vi "Continuous Volume Demo.vi"() -> ()   [LabVIEW 2012]
uses:
  LabVIEW/user.lib/SpectralRadar.llb/Data Analyzation Selection.ctl
  LabVIEW/user.lib/SpectralRadar.llb/Device Camera Preset Selection.ctl
  LabVIEW/user.lib/SpectralRadar.llb/Processing Flag Selection.ctl
  LabVIEW/user.lib/SpectralRadar.llb/Normal Direction Selection.ctl
  LabVIEW/user.lib/SpectralRadar.llb/set Apodized Spectrum Output.vi
  LabVIEW/user.lib/SpectralRadar.llb/set Scan Output.vi
  LabVIEW/user.lib/SpectralRadar.llb/display Data 2D.vi
  LabVIEW/user.lib/SpectralRadar.llb/OCT Device.lvclass
  LabVIEW/user.lib/SpectralRadar.llb/Probe.lvclass
  LabVIEW/user.lib/SpectralRadar.llb/Processing.lvclass
  LabVIEW/user.lib/SpectralRadar.llb/Raw Data.lvclass
  LabVIEW/user.lib/SpectralRadar.llb/Data.lvclass
  LabVIEW/user.lib/SpectralRadar.llb/Scan Pattern.lvclass
panel:
  in  "Slice vs. Process":bool
  in  "Data Analyzation Selection":T1
  out "B-Scan Data":dbl[][](graph)
  in  "Index":i32(slide) min=0 max=1023 step=1 scale=0.0..1023.0
  in  "stop":bool
  out "En-Face Data":dbl[][](graph)
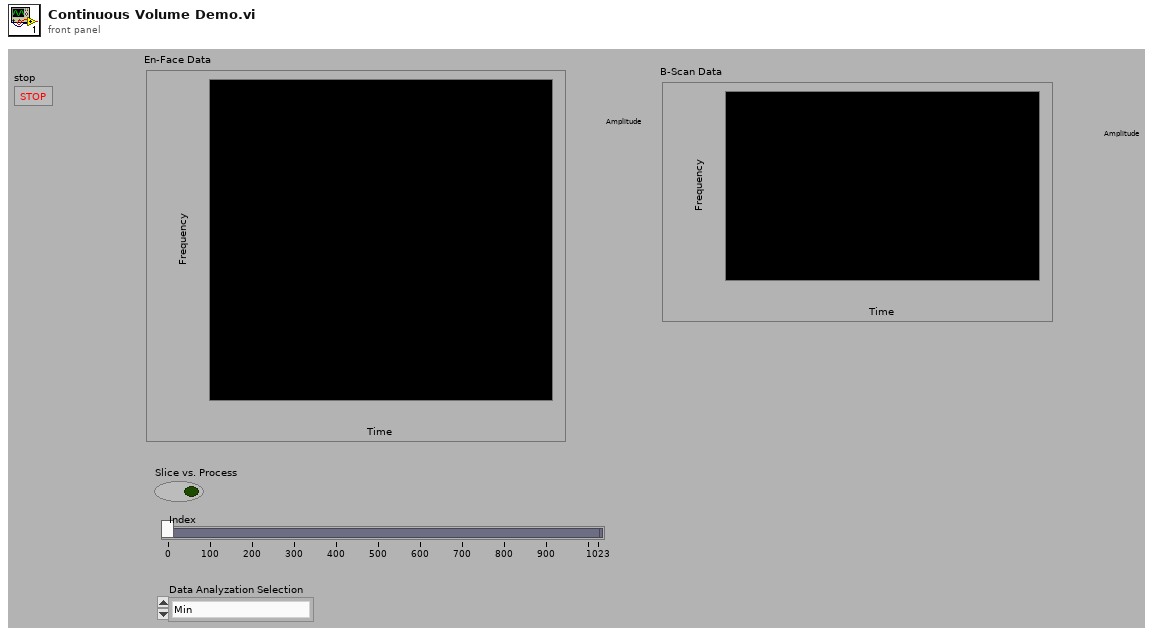
[diagram p1: front panel]
types:
  T1 = typedef "Data.lvclass/Data Analyzation Selection.ctl" = enum16{"Min", "Mean", "Max"}
  T2 = typedef "Processing.lvclass/Processing Flag Selection.ctl" = enum16{"Use Offset Errors", "Remove DC Spectrum", "Remove Advanced DC Spectrum", "Use Apodization", "Use Scan For Apodization", "Filter Undersampled Signals", "Use Dispersion Compensation", "Use Dechirp", "Use Extended Adjust", "Full Range Output", "Filter DC", "Autocorrelation Compensation", "DEFR", "Only Windowing", "Remove Fixed Pattern"}
  T3 = typedef "OCT Device.lvclass/Device Camera Preset Selection.ctl" = enum16{"Default", "Preset 1", "Preset 2", "Preset 3"}
  T4 = enum16{"Asynchronous Continuous", "Asynchronous Finite", "Synchronous"}
  T5 = typedef "Data.lvclass/Normal Direction Selection.ctl" = enum16{"Direction 1", "Direction 2", "Direction 3"}
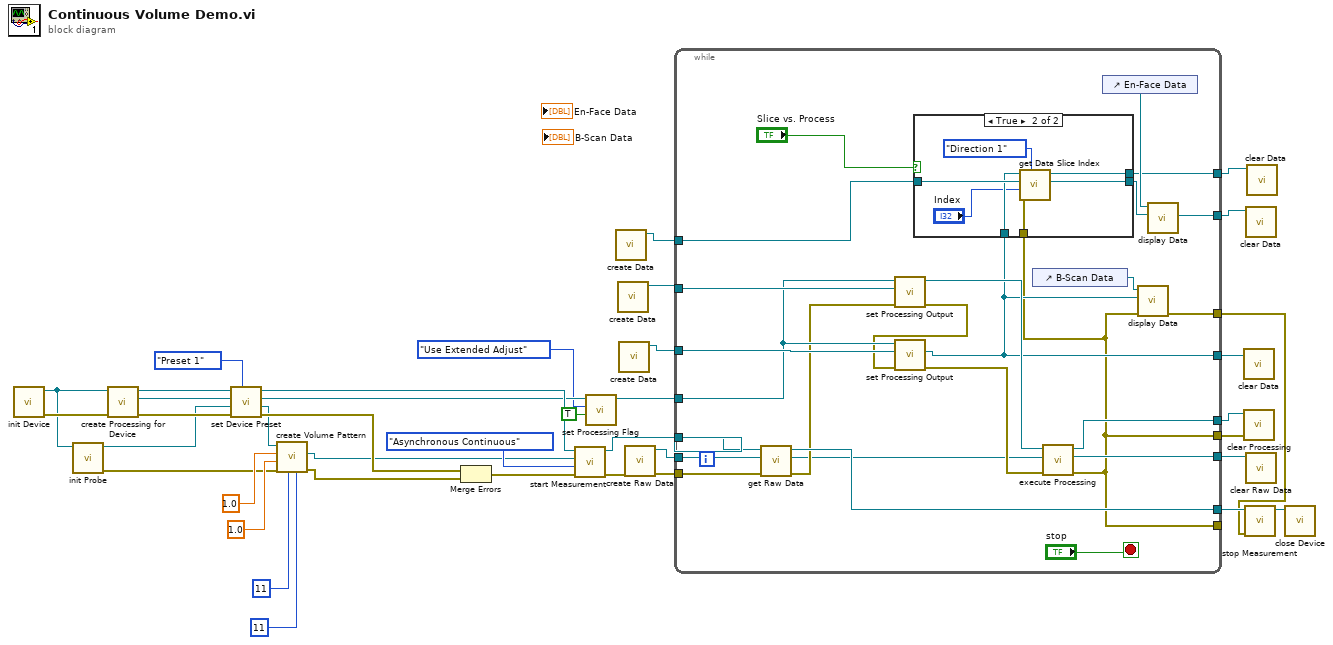
[diagram p0: block diagram]
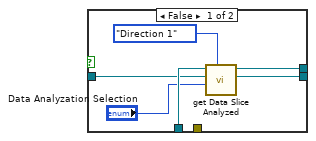
[diagram p2: hidden frame]
diagram:
  n1 = call "init Device.vi"() -> ("error out"=w38:errorcluster, "OCTDevice"=w30:refnum<class "OCT Device.lvclass">)  [unwired: 6 in]
  n2 = call "init Probe.vi"("OCT Device"=w30) -> ("error out"=w16:errorcluster, "GalvoControl"=w25:refnum<class "Probe.lvclass">)  [unwired: 5 in]
  n3 = call "create Processing for Device.vi"("error in (no error)"=w38, "OCTDevice"=w30) -> ("error out"=w35:errorcluster, "Processing"=w23:refnum<class "Processing.lvclass">, "OCTDevice"=w26:refnum<class "OCT Device.lvclass">)  [unwired: 3 in]
  n4 = call "set Device Preset.vi"("Numeric"=Device_Camera_Preset_Selection."Preset 1" ("Device Camera Preset Selection"), "Probe"=w25, "Processing"=w23, "OCTDevice"=w26) -> ("Probe 2"=w21:refnum<class "Probe.lvclass">, "Processing"=w13:refnum<class "Processing.lvclass">, "OCTDevice out"=w24:refnum<class "OCT Device.lvclass">)  [unwired: 2 in, 1 out]
  n5 = call "create Volume Pattern.vi"("Size Y"=11, "Size X"=11, "error in (no error)"=w16, "Range Y"=1.0, "Range X"=1.0, "Probe"=w21) -> ("error out"=w15:errorcluster, "Scan Pattern"=w14:refnum<class "Scan Pattern.lvclass">)  [unwired: 1 in, 1 out]
  n6 = Merge Errors(w35, w15) -> (w36:errorcluster)
  n7 = call "start Measurement.vi"("error in (no error)"=w36, "Acquisition Type"=T4."Asynchronous Continuous", "Scan Pattern"=w14, "OCTDevice"=w24) -> ("error out"=w33:errorcluster, "OCTDevice"=w27:refnum<class "OCT Device.lvclass">)  [unwired: 1 in, 1 out]
  n8 = call "set Processing Flag.vi"("Flag"=TRUE, "Processing Flag Selection"=Processing_Flag_Selection."Use Extended Adjust", "Processing"=w13) -> ("Processing"=w12:refnum<class "Processing.lvclass">)  [unwired: 3 in, 1 out]
  n9 = call "create Data.vi"() -> ("Data"=w1:refnum<class "Data.lvclass">)  [unwired: 6 in, 1 out]
  n10 = call "create Data.vi"() -> ("Data"=w2:refnum<class "Data.lvclass">)  [unwired: 6 in, 1 out]
  n11 = call "create Data.vi"() -> ("Data"=w3:refnum<class "Data.lvclass">)  [unwired: 6 in, 1 out]
  n12 = call "create Raw Data.vi"("error in (no error)"=w33) -> ("error out"=w32:errorcluster, "Raw Data"=w34:refnum<class "Raw Data.lvclass">)  [unwired: 5 in]
  n13 = while {
    tunnel: w34 -> [w62]
    tunnel: w27 -> [w63]
    tunnel: w32 -> [w61]
    tunnel: w12 -> [w58]
    tunnel: w3 -> [w60]
    tunnel: w2 -> [w59]
    tunnel: [w53] -> w31
    tunnel: [w52] -> w8
    tunnel: [w42] -> w6
    tunnel: [w51] -> w29
    tunnel: [w41] -> w7
    tunnel: [w41] -> _
    tunnel: w1 -> [w47]
    tunnel: [w46] -> w5
    tunnel: [w44] -> w4
    tunnel: [w39] -> w9
    stop <- "stop" stop-if-true
    n14 = call "get Raw Data.vi"("error in (no error)"=w61, "RawData in"=w62, "OCTDevice in"=w63) -> ("error out"=w50:errorcluster, "RawData out"=w48:refnum<class "Raw Data.lvclass">, "OCTDevice out"=w51:refnum<class "OCT Device.lvclass">)  [unwired: 2 in]
    n15 = call-poly "set Processing Output.vi"("error in (no error)"=w50, "Data"=w59, "Processing"=w58) -> ("error out"=w56:errorcluster, "Processing"=w57:refnum<class "Processing.lvclass">)  [unwired: 2 in, 1 out]
    n16 = call-poly "set Processing Output.vi"("error in (no error)"=w56, "Data"=w60, "Processing"=w58) -> ("error out"=w55:errorcluster, "Data"=w42:refnum<class "Data.lvclass">)  [unwired: 2 in, 1 out]
    n17 = control-ref of="B-Scan Data"() -> (w43:refnum<vi>)
    n18 = call "execute Processing.vi"("error in (no error)"=w55, "Raw Data"=w48, "Processing"=w57) -> ("error out"=w41:errorcluster, "Raw Data"=w53:refnum<class "Raw Data.lvclass">, "Processing"=w52:refnum<class "Processing.lvclass">)  [unwired: 2 in]
    n19 = case shown="True" "Slice vs. Process" {
      tunnel: w47 -> [w68 w76]
      tunnel: [w64 w74] -> w45
      tunnel: [w65 w73] -> w44
      tunnel: w42 -> [w69 w72]
      tunnel: w41 -> [_ w71]
      frame False {
        n20 = call "get Data Slice Analyzed.vi"("Normal Direction"=Normal_Direction_Selection."Direction 1", "Data Analyzation Selection"="Data Analyzation Selection", "Slice"=w68, "Data"=w69) -> ("Slice"=w64:refnum<class "Data.lvclass">, "Data"=w65:refnum<class "Data.lvclass">)  [unwired: 3 in, 1 out]
      }
      frame True {
        n21 = call "get Data Slice Index.vi"("Normal Direction"=Normal_Direction_Selection."Direction 1", "error in (no error)"=w71, "Index"="Index", "Slice"=w76, "Data"=w72) -> ("Slice"=w74:refnum<class "Data.lvclass">, "Data"=w73:refnum<class "Data.lvclass">)  [unwired: 2 in, 1 out]
      }
    }
    n22 = control-ref of="En-Face Data"() -> (w54:refnum<vi>)
    n23 = call-poly "display Data.vi"("error in (no error)"=w41, "Data in"=w42, "IntGraph Refnum"=w43) -> ("error out"=w39:errorcluster)  [unwired: 2 in, 2 out]
    n24 = call-poly "display Data.vi"("Data in"=w45, "IntGraph Refnum"=w54) -> ("Data out"=w46:refnum<class "Data.lvclass">)  [unwired: 3 in, 2 out]
  }
  n25 = call "clear Data.vi"("Data"=w6) -> ()  [unwired: 6 in, 1 out]
  n26 = call "clear Processing.vi"("error in (no error)"=w7, "Processing"=w8) -> ()  [unwired: 5 in, 1 out]
  n27 = call "stop Measurement.vi"("error in (no error)"=w9, "OCTDevice"=w29) -> ("OCTDevice"=w28:refnum<class "OCT Device.lvclass">)  [unwired: 4 in, 1 out]
  n28 = call "clear Data.vi"("Data"=w5) -> ()  [unwired: 6 in, 1 out]
  n29 = call "clear Raw Data.vi"("Raw Data"=w31) -> ()  [unwired: 6 in, 1 out]
  n30 = call "clear Data.vi"("Data"=w4) -> ()  [unwired: 6 in, 1 out]
  n31 = call "close Device.vi"("OCTDevice"=w28) -> ()  [unwired: 6 in, 1 out]
